vi "SR1.read data.vi"(0 "i ref in":refnum<vi>, 5 "error in (no error)":errorcluster) -> (14 "i ref out":refnum<vi>, 16 "Output Waveform":T1, 19 "error out":errorcluster)   [LabVIEW 2014, in "SR1.lvlib"]
doc: "gets the data in binary format from the SR1. The data format is a waveform flattened to string.\n\nThis method performs a sequence of the following methods.\n\n- stop scan\n- read bin data\n- start scan"
uses:
  SR1.lvlib
  CS_Core/CSSystem/CoreDefs/CoreDefs.rawDataType.ctl
  CSlibraries/UtilityLib/UtilityLib.valueStatus.ctl
  CS_Core/CSApplicationBaseClasses/NABase/NABase.directionType.ctl
  CS_Core/CSApplicationBaseClasses/NABase/NABase.serviceType.ctl
  CS_Core/CSApplicationBaseClasses/NABase/NABase.statusType.ctl
  CSlibraries/UtilityLib/UtilityLib.lvlib
  CS_Core/CSApplicationBaseClasses/NABase/NABase.lvlib
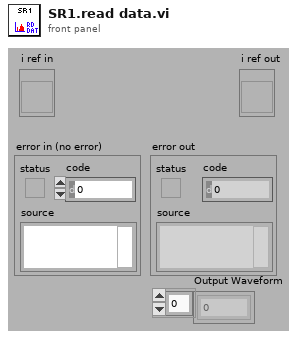
[diagram p1: front panel]
types:
  T1 = typedef "CoreDefs.rawDataType.ctl" = i8[]
  T2 = typedef "NABase.lvlib/NABase.serviceType.ctl" = enum16{"StartFreq", "NofLines", "FreqSpan", "status", "triggerLevel", "triggerSlope", "TimeRecDur", "NofStoredData"}
  T3 = typedef "NABase.lvlib/NABase.directionType.ctl" = enum16{"unknown", "update actual value", "update nominal value", "update both"}
  T4 = typedef "UtilityLib.lvlib/UtilityLib.valueStatus.ctl" = enum16{"no info available", "stand by/off", "on", "warning", "alarm/malfunction", "not implemented", "user action required", "important information", "system default", "control default", "indicator default", "button default"}
  T5 = typedef "NABase.lvlib/NABase.statusType.ctl" = i32
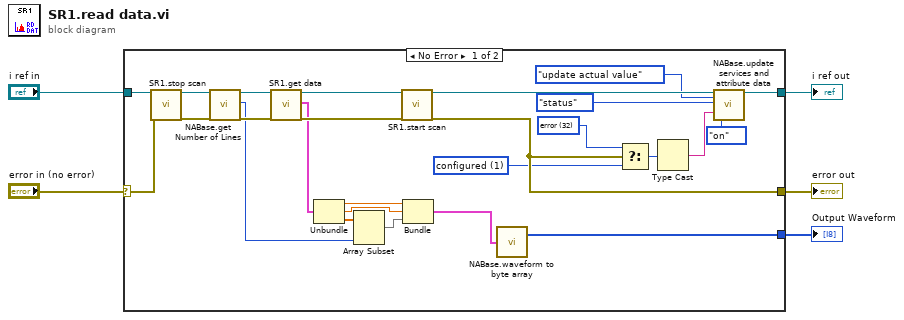
[diagram p0: block diagram]
diagram:
  n1 = case shown="No Error" "error in (no error)" {
    selector: "error in (no error)" -> [w26 w32]
    tunnel: "i ref in" -> [w31 w33]
    tunnel: [w19 w32] -> w4
    tunnel: [w20 w33] -> w3
    tunnel: [w25 _] -> w2
    frame No Error {
      w15 = T5 1 items=["unknown"=0, "configured"=1, "error"=32] ("service")
      w16 = T5 32 items=["unknown"=0, "configured"=1, "error"=32] ("service")
      n2 = call "SR1.stop scan.vi"("i ref in"=w31, "error in (no error)"=w26) -> ("i ref out"=w28:refnum<vi>, "error out"=w27:errorcluster)  [unwired: 16 in]
      n3 = call "NABase.get Number of Lines.vi"("i ref in"=w28, "error in (no error)"=w27) -> ("i ref out"=w30:refnum<vi>, "NofLines"=w10:i32, "error out"=w29:errorcluster)  [unwired: 15 in]
      n4 = call "SR1.get data.vi"("i ref in"=w30, "error in (no error)"=w29) -> ("i ref out"=w14:refnum<vi>, "Output Waveform"=w12:cluster{dbl, dbl, dbl[]}, "error out"=w13:errorcluster)  [unwired: 15 in]
      n5 = Unbundle(w12) -> (w8:dbl, w7:dbl, w11:dbl[])
      n6 = Array Subset(array=w11, length=w10) -> (w9:dbl[])  [unwired: 1 in]
      n7 = call "SR1.start scan.vi"("i ref in"=w14, "error in (no error)"=w13) -> ("i ref out"=w21:refnum<vi>, "error out"=w19:errorcluster)  [unwired: 16 in]
      n8 = Bundle(w8, w7, w9) -> (w6:cluster{dbl, dbl, dbl[]})  [unwired: 1 in]
      n9 = call "NABase.waveform to byte array.vi"("Waveform"=w6) -> ("byteArray out"=w25:T1)  [unwired: 1 out]
      n10 = Select(t=w16, s=w19, f=w15) -> (s? t:f=w22:T5)
      n11 = Type Cast(x=w22) -> (*(type *) &x=w23:string)  [unwired: 1 in]
      n12 = call "NABase.update services and attribute data.vi"("i ref in"=w21, "direction"=NABase.directionType."update actual value", "service"=NABase.serviceType."status", "value"=w23, "quality"=UtilityLib.valueStatus."on") -> ("i ref out"=w20:refnum<vi>)  [unwired: 12 in, 2 out]
    }
    frame Error {
    }
  }
  "error out" <- w4
  "i ref out" <- w3
  "Output Waveform" <- w2
